vi "Configure Digital Channels.vi"(0 "VISA resource name":refnum<visa-resource-name>, 1 "Digital Channels":u16(ring) items=["0", "2", "4", "6", "8", "10", "12", "14", "16", "18", "20", "22", "24", "26", "28", "30", "32"], 2 "Voltage Level Selection":u8(ring) items=["Value", "Minimum", "Maximum", "Default"], 3 "error in (no error)":errorcluster, 4 "Skew Selection":u8(ring) items=["Value", "Minimum", "Maximum", "Default"], 5 "Digital Pod (0: Digital Pod A)":u16(ring) items=["Pod A", "Pod B", "Pod C", "Pod D"], 7 "Voltage Level (V)":dbl=1.0, 8 "Skew (s)":dbl) -> (6 "VISA resource name out":refnum<visa-resource-name>, 9 "error out":errorcluster)   [LabVIEW 2020, in "Active Technologies AWG3000.lvlib"]
uses:
  Active Technologies AWG3000.lvlib
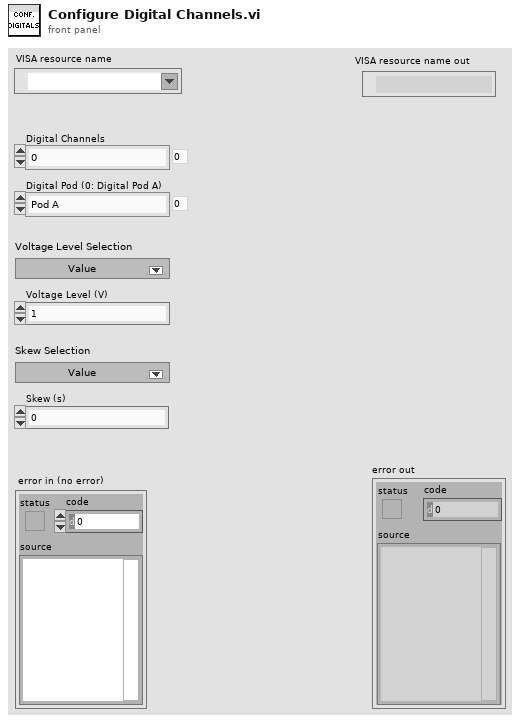
[diagram p1: front panel]
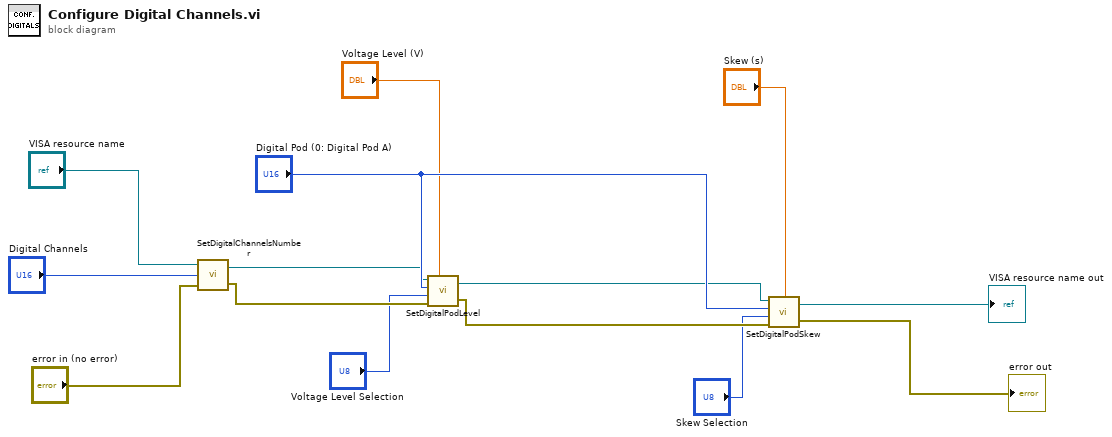
[diagram p0: block diagram]
diagram:
  n1 = call "SetDigitalChannelsNumber.vi"("error in (no error)"="error in (no error)", "Digital Channels"="Digital Channels", "VISA resource name"="VISA resource name") -> ("error out"=w6:errorcluster, "VISA resource name out"=w7:refnum<visa-resource-name>)
  n2 = call "SetDigitalPodLevel.vi"("VISA resource name"=w7, "Digital Pod (0: Digital Pod A)"="Digital Pod (0: Digital Pod A)", "Selection"="Voltage Level Selection", "error in (no error)"=w6, "Voltage Level (V)"="Voltage Level (V)") -> ("VISA resource name out"=w4:refnum<visa-resource-name>, "error out"=w3:errorcluster)
  n3 = call "SetDigitalPodSkew.vi"("VISA resource name"=w4, "Digital Pod (0: Digital Pod A)"="Digital Pod (0: Digital Pod A)", "Selection"="Skew Selection", "error in (no error)"=w3, "Skew (s)"="Skew (s)") -> ("VISA resource name out"=→"VISA resource name out":refnum<visa-resource-name>, "error out"=→"error out":errorcluster)
